vi "Control Experiment Class from JSON.vi"(8 "error in (no error)":errorcluster, 10 "JSON":string, 11 "Control Experiment in":refnum<class "Control Experiment.lvclass">) -> (0 "error out":errorcluster, 3 "Control Experiment out":refnum<class "Control Experiment.lvclass">)   [LabVIEW 2019, in "Control Experiment.lvclass"]
uses:
  Control Experiment.lvclass
  Typedefs/Control Experiment FGV.JSON--cluster.ctl
  Typedefs/Experiment Description--cluster.ctl
  Typedefs/Instruments--cluster.ctl
  Typedefs/Instrument Types--enum.ctl
  Typedefs/Wiring Description--cluster.ctl
  Control Experiment.lvclass/Control Experiment.ctl
  <userlib>/LevyLab/Instrument Framework/Instrument/Instrument.lvclass
  <userlib>/LevyLab/Instrument Framework/Instrument/Instrument.lvclass/Instrument.ctl
  dbafe0ef-e718-4924-8c3c-ddc720cb6ca1.vi
  <vilib>/JDP Science/JSONtext/JSON text to Variant.vi
  <vilib>/JDP Science/JSONtext/LVClass Serializer/JSONtext LVClass Serializer.lvclass
  Attributes/Instrument Attributes.lvlib
  C:/Program Files (x86)/National Instruments/LabVIEW 2019/vi.lib/JKI/JKI SMO/SMO/SMO.lvclass
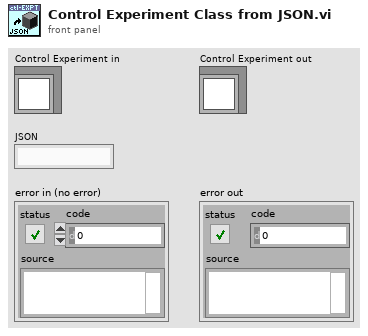
[diagram p1: front panel]
types:
  T1 = typedef "Control Experiment.lvclass/Control Experiment FGV.JSON--cluster.ctl" = cluster{"json":string, "Experiment":T2, "Wiring Configuration":T5}
  T2 = typedef "Control Experiment.lvclass/Experiment Description--cluster.ctl" = cluster{"User":string, "Device":string, "Device Path":path, "Device Description":string, "Experiment Path":path, "Experiment Description":string, "Instrument":string, "Instruments":T3[], "Sweep":cluster{"key":string, "value":variant}[]}
  T3 = typedef "Control Experiment.lvclass/Instruments--cluster.ctl" = cluster{"class path":path, "Address":string, "Type":T4}
  T4 = typedef "Control Experiment.lvclass/Instrument Types--enum.ctl" = enum16{"DAQ", "Amplifier", "Temperature", "Magnet", "Rotator", "Level", "Capacitance", "Delay Line", "Strain Cell", "VNA", "Source"}
  T5 = typedef "Control Experiment.lvclass/Wiring Description--cluster.ctl" = cluster{"Lockin Ch":i32[], "KH":cluster{"Electrodes":string[], "Labels":string[]}, "not KH":cluster{"Electrodes":string[], "Labels":string[]}}
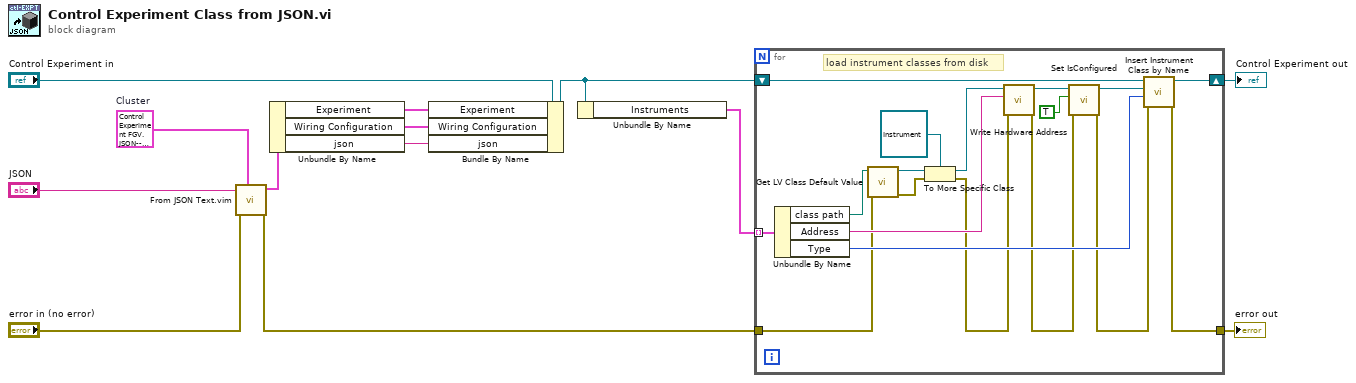
[diagram p0: block diagram]
diagram:
  w2 = T1 {"json"="", "Experiment"={"User"="", "Device"="", "Device Path"=path "", "Device Description"="", "Experiment Path"=path "", "Experiment Description"="", "Instrument"="", "Instruments"=[], "Sweep"=[]}, "Wiring Configuration"={"Lockin Ch"=[], "KH"={"Electrodes"=[], "Labels"=[]}, "not KH"={"Electrodes"=[], "Labels"=[]}}}  # Cluster
  n1 = call "From JSON Text.vim"("Data Type and Default Value"=w2, "error in (no error)"="error in (no error)", "JSON"="JSON") -> ("error out"=w10:errorcluster, "Data out"=w5:T1)  [unwired: 7 in]
  n2 = Unbundle By Name(w5) -> ("Experiment"=w8:T2, "Wiring Configuration"=w7:T5, "json"=w3:string)
  n3 = Bundle By Name(cluster="Control Experiment in", "Experiment"=w8, "Wiring Configuration"=w7, "json"=w3) -> (w1:refnum<class "Control Experiment.lvclass">)
  n4 = Unbundle By Name(w1) -> ("Instruments"=w4:T3[])
  n5 = for {
    tunnel: w4 -> [w31] mode=indexing
    tunnel: w10 -> [w22]
    tunnel: [w25] -> w12
    shift-right: [w26] -> w6
    shift-left: w1 -> [w27]
    # "load instrument classes from disk"
    n6 = Unbundle By Name(w31) -> ("class path"=w21:path, "Address"=w24:string, "Type"=w23:T4)
    n7 = call <vilib>:"Get LV Class Default Value.vi"("error in (no error)"=w22, "class path"=w21) -> ("error out"=w28:errorcluster, "object"=w30:refnum<class>)  [unwired: 8 in]
    n8 = To More Specific Class(target class=refnum<class "Instrument.lvclass"> refnum ("Instrument in"), reference=w30, error in=w28) -> (specific class reference=w19:refnum<class "Instrument.lvclass">, error out=w20:errorcluster)
    n9 = call <userlib>:"Write Hardware Address.vi"("error in (no error)"=w20, "Address"=w24, "Instrument in"=w19) -> ("error out"=w16:errorcluster, "Instrument out"=w18:refnum<class "Instrument.lvclass">)  [unwired: 7 in]
    n10 = call "Set IsConfigured.vi"("error in (no error)"=w16, "IsConfigured?"=TRUE, "SMO"=w18) -> ("error out"=w15:errorcluster, "SMO out"=w17:refnum<class "Instrument.lvclass">)  [unwired: 7 in]
    n11 = call "Insert Instrument Class by Name.vi"("error in (no error)"=w15, "Type"=w23, "Instrument in"=w17, "Control Experiment in"=w27) -> ("error out"=w25:errorcluster, "Control Experiment out"=w26:refnum<class "Control Experiment.lvclass">)  [unwired: 4 in, 2 out]
  }
  "Control Experiment out" <- w6
  "error out" <- w12
